vi "sub_get_array_element.vi"(8 "error in (no error)":errorcluster, 10 "Desired element":dbl=2.5 format="%#_13g", 11 "Array":dbl[](array[numeric])) -> (0 "error out":errorcluster, 2 "New index":i32)   [LabVIEW 2016]
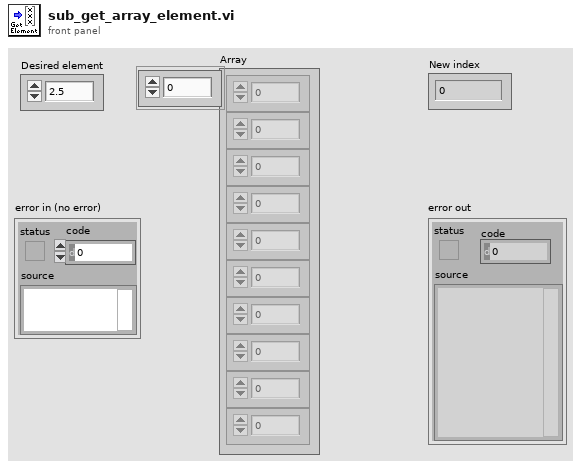
[diagram p1: front panel]
types:
  T1 = enum16{"Left Button", "Center Button", "Right Button", "Window Close"}
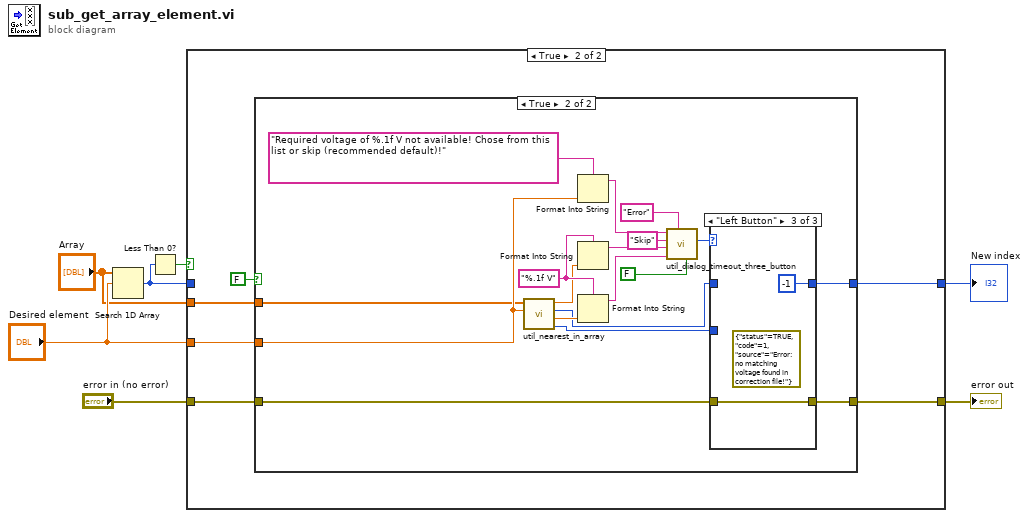
[diagram p0: block diagram]
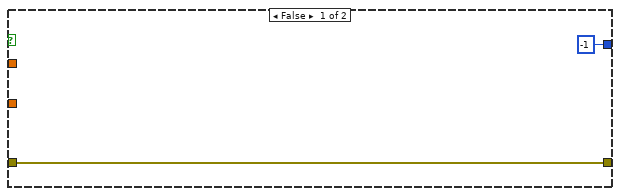
[diagram p3: hidden frame]
diagram:
  n1 = Search 1D Array(1D array="Array", element="Desired element") -> (index of element=w5:i32)  [unwired: 1 in]
  n2 = Less Than 0?(x=w5) -> (x < 0?=w7:bool)
  n3 = case shown="True" w7 {
    tunnel: w5 -> [w9 _]
    tunnel: [w9 w13] -> w6
    tunnel: "Array" -> [_ w14]
    tunnel: "Desired element" -> [_ w15]
    tunnel: "error in (no error)" -> [w8 w12]
    tunnel: [w8 w11] -> w1
    frame False {
    }
    frame True {
      n4 = case shown="True" FALSE {
        tunnel: w15 -> [_ w33]
        tunnel: w14 -> [_ w32]
        tunnel: [-1 ("2nd closest index") w27] -> w13
        tunnel: w12 -> [w17 w26]
        tunnel: [w17 w25] -> w11
        frame False {
        }
        frame True {
          w34 = "%.1f V" ("format string")
          n5 = call "util_nearest_in_array.vi"("desired element"=w33, "1D Array"=w32) -> ("2nd closest index"=w29:i32, "2nd closest element"=w30:dbl, "closest index"=w28:i32, "closest element"=w31:dbl)  [unwired: 6 in]
          n6 = Format Into String(format string="Required voltage of %.1f V not available! Chose from this list or skip (recommended default)!" ("Window Title (\"\")"), w33) -> (resulting string=w23:string)  [unwired: 2 in, 1 out]
          n7 = Format Into String(format string=w34, w31) -> (resulting string=w19:string)  [unwired: 2 in, 1 out]
          n8 = Format Into String(format string=w34, w30) -> (resulting string=w20:string)  [unwired: 2 in, 1 out]
          n9 = call "util_dialog_timeout_three_button.vi"("Allow user to close window? (TRUE)"=FALSE, "Window Title (\"\")"="Error" ("Window Title (\"\")"), "Right Button Text (\"Cancel\")"=w20, "Center Button Text (\"No\")"=w19, "Default Button Text (\"Yes\")"="Skip" ("Default Button Text (\"Yes\")"), "message"=w23) -> ("Which Button?"=w21:T1)  [unwired: 5 in]
          n10 = case shown="\"Left Button\"" w21 {
            tunnel: w28 -> [w37 _ _]
            tunnel: w29 -> [_ w39 _]
            tunnel: [w37 w39 -1] -> w27
            tunnel: w26 -> [w36 w38 w40]
            tunnel: [w36 w38 w40] -> w25
            frame "Center Button", Default {
            }
            frame "Right Button" {
            }
            frame "Left Button" {
              (unwired) errorcluster {"status"=TRUE, "code"=1, "source"="Error: no matching voltage found in correction file!"} ("error constant")
            }
          }
        }
      }
    }
  }
  "New index" <- w6
  "error out" <- w1
